vi "RealTime.vi"() -> ()   [LabVIEW 2019]
uses:
  ByteGSAPIBase/LimsTestStep/acquisitions.ctl
  <vilib>/Bytelabs/ByteChannelsSetting/ChannelSettingsLib/ChannelsRepos/ChannelsRepoXML/ChannelsRepoXML.lvclass
  C:/Program Files (x86)/National Instruments/LabVIEW 2019/vi.lib/Bytelabs/ByteChannelsSetting/ChannelSettingsLib/ChannelsRepos/ChannelsRepoBase/ChannelsRepoBase.lvclass
  TypeDef/ChannelInfo.ctl
  ByteGSAPIBase/ByteGSAPIBase.lvclass
  TypeDef/TCPMessage.ctl
  <vilib>/Bytelabs/ByteChannelsSetting/ChannelSettingsLib/ChannelsClasses/ChannelBase/ChannelBase.lvclass/ChannelBase.ctl
  ByteGSAPIBase/UpdateChannelsList/fields.ctl
  ByteGSAPIBase/TypeDef/Step.ctl
  ByteGSAPIBase/TypeDef/Asset.ctl
  <vilib>/Utility/xml.llb/Write to XML File(string).vi
  bytetcp/TCPLib/TCP_Class/TCP.lvclass
  <vilib>/Bytelabs/ByteSimpleQ/ByteSimpleQ/ByteSimpleQ.lvlib
  <vilib>/Bytelabs/ByteChannelsSetting/ChannelSettingsLib/ChannelsRepos/ChannelsRepoBase/ChannelsRepoBase.lvclass
  <vilib>/Bytelabs/ByteChannelsSetting/ChannelSettingsLib/ChannelsClasses/ChannelBase/ChannelBase.lvclass
panel:
  out "error out":errorcluster
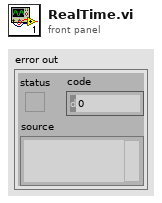
[diagram p1: front panel]
types:
  T1 = typedef "ChannelInfo.ctl" = cluster{"Tag":string, "HW Resource":string, "Raw":dbl}
  T2 = typedef "ByteGSWebAPI.lvlib/ByteGSAPIBase.lvclass/acquisitions.ctl" = cluster{"tags":cluster{"step_id":i32, "test_slug":string, "asset_slug":string}, "acquisitions":cluster{"timestamp":string, "fields":cluster{"name":string, "value":dbl}[]}[]}
  T3 = cluster{"queue out":refnum<queue>, "Acquisitions":T2, "Info":T1[], "TCP_Class":refnum<class "TCP.lvclass">, "Continous?":bool, "Duration":dbl, "ByteGSAPIBase in":refnum<class "ByteGSAPIBase.lvclass">}
  T4 = cluster{"ByteGSAPIBase in":refnum<class "ByteGSAPIBase.lvclass">, "TCP_Class":refnum<class "TCP.lvclass">, "ChannelsRepoBase out":refnum<class "ChannelsRepoXML.lvclass">, "queue out":refnum<queue>}
  T5 = cluster{"ChannelsRepoBase out":refnum<class "ChannelsRepoXML.lvclass">, "channels":string[], "Duration":dbl, "id":i32, "prova.slug":string, "Continous?":bool, "ByteGSAPIBase in":refnum<class "ByteGSAPIBase.lvclass">}
  T6 = cluster{"timestamp":string, "fields":cluster{"name":string, "value":dbl}[]}
  T7 = typedef "TCPMessage.ctl" = cluster{"Message":string, "Data":variant}
  T8 = cluster{"timestamp":string, "fields":cluster{"name":string, "value":dbl}[]}[]
  T9 = typedef "ByteGSWebAPI.lvlib/ByteGSAPIBase.lvclass/fields.ctl" = cluster{"asset_slug":string, "fields":string[]}
  T10 = typedef "ByteGSWebAPI.lvlib/ByteGSAPIBase.lvclass/Step.ctl" = cluster{"id":i32, "descrizione":string, "prova":cluster{"slug":string}, "assets":T11[], "criterio_accettazione":string, "valore_criterio_accettazione_max":dbl, "valore_criterio_accettazione_min":dbl, "udm_criterio_accettazione":string, "duration_prova":string, "udm_duration_prova":string, "valore_prova":dbl, "ordine":i32, "user":i32, "link_automation":string, "instruction_automation":string, "data_completamento_checklist":timestamp, "outcome":bool, "step_type":string, "channels":string[]}
  T11 = typedef "ByteGSWebAPI.lvlib/ByteGSAPIBase.lvclass/Asset.ctl" = cluster{"descrizione":string, "slug":string, "id":i32}
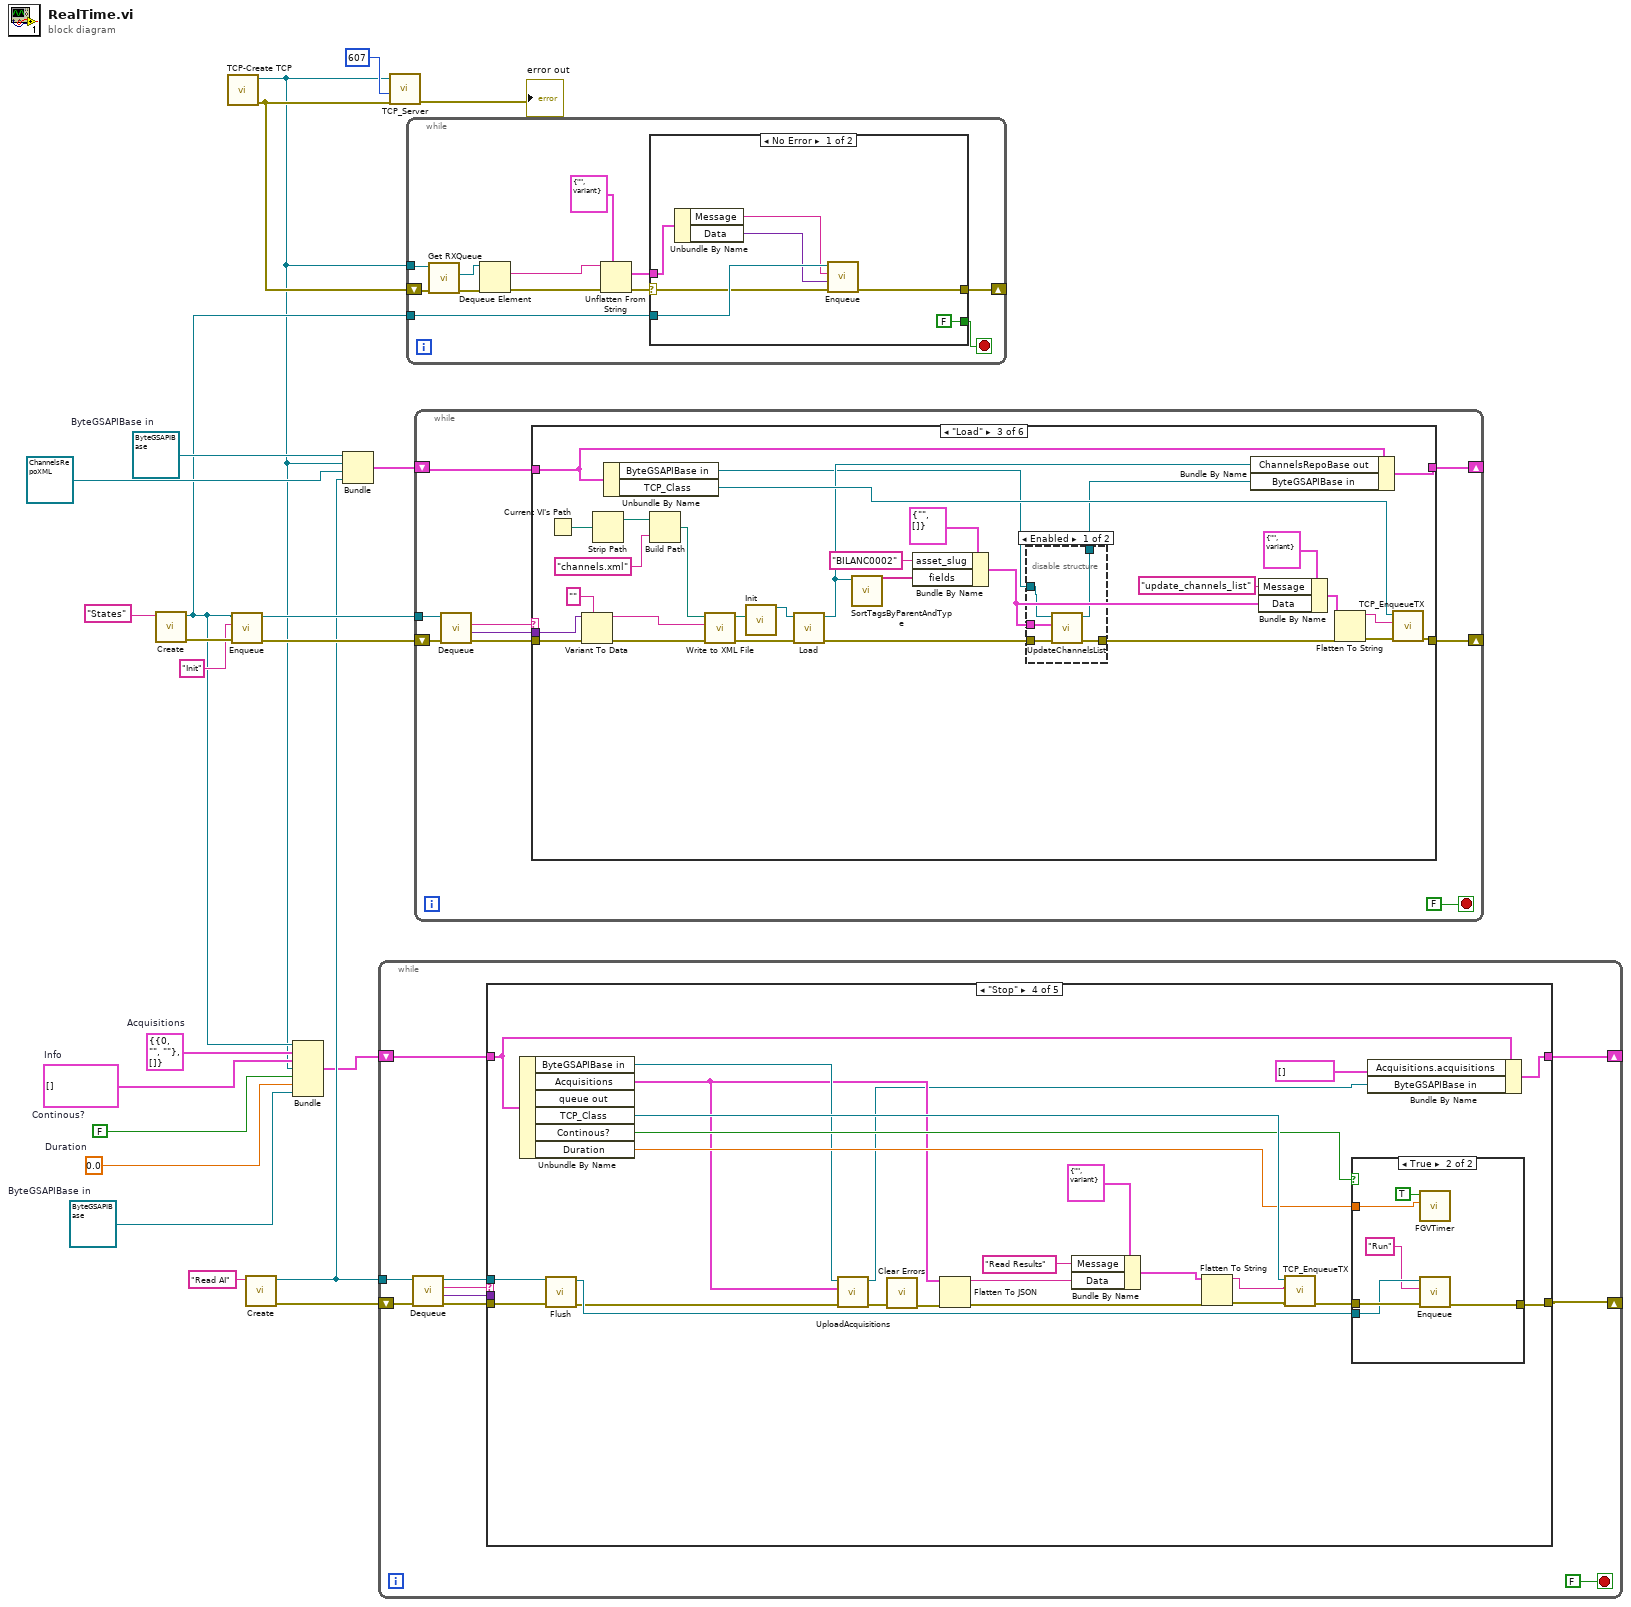
[diagram p0: block diagram]
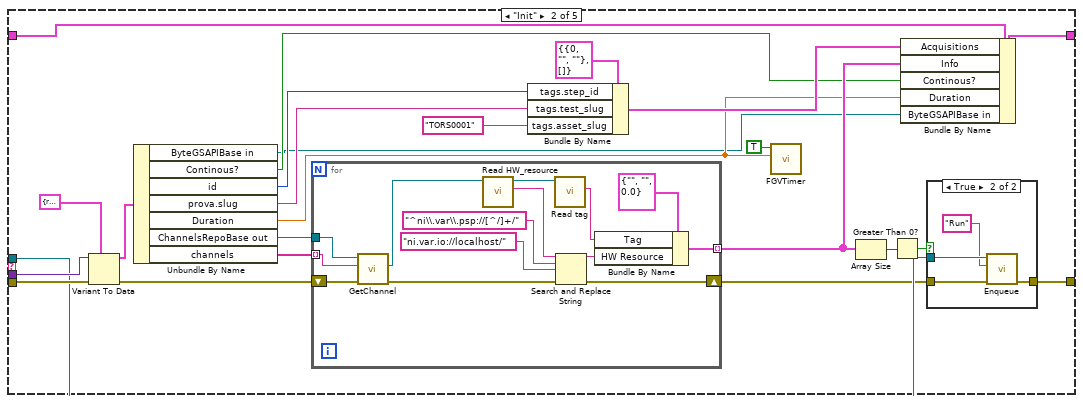
[diagram p3: hidden frame]
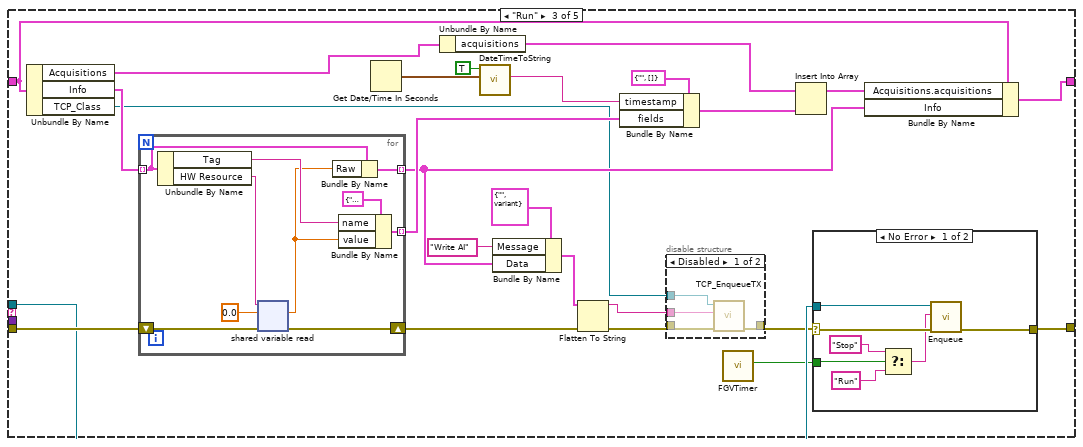
[diagram p5: hidden frame]
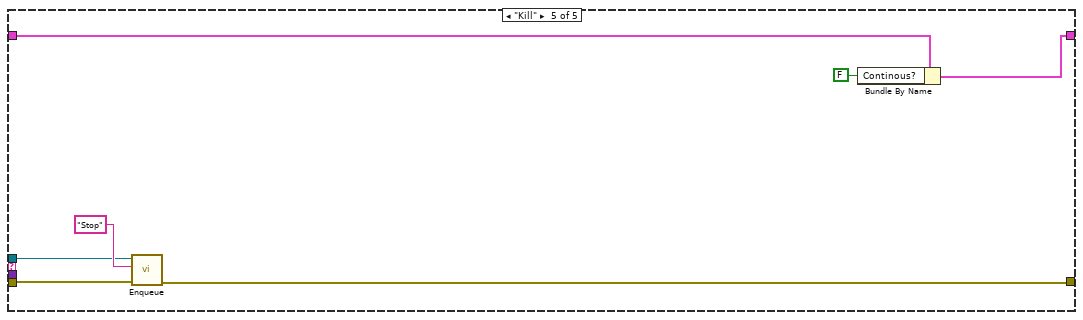
[diagram p9: hidden frame]
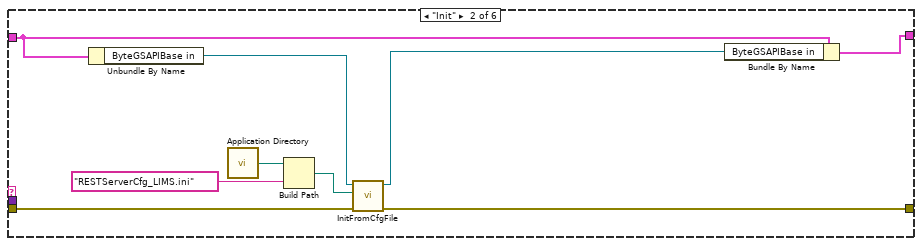
[diagram p11: hidden frame]
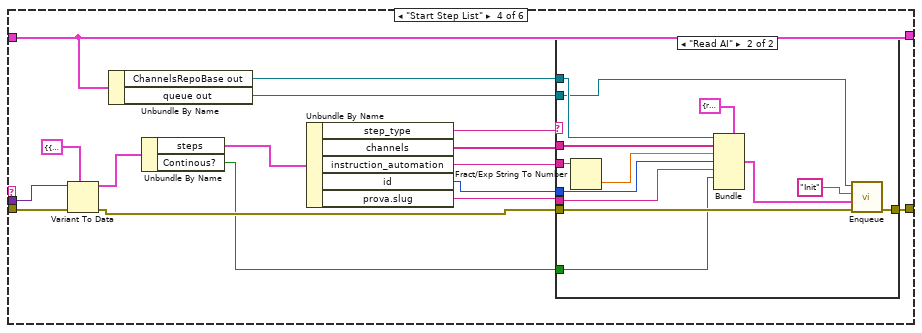
[diagram p13: hidden frame]
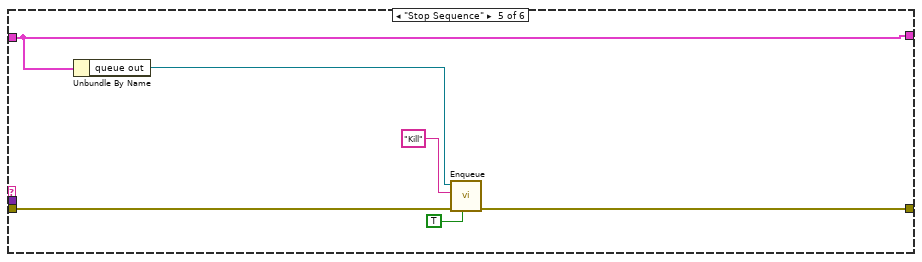
[diagram p15: hidden frame]
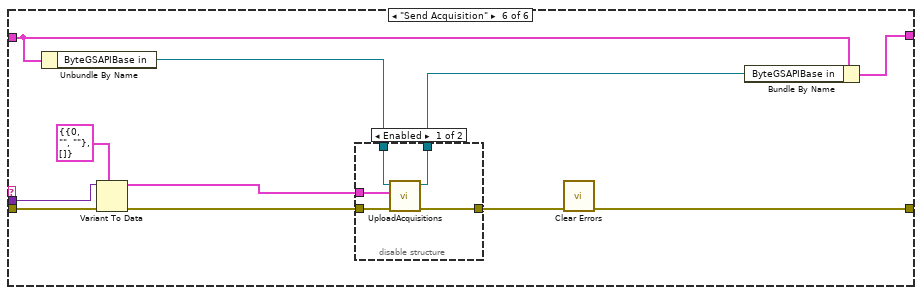
[diagram p16: hidden frame]
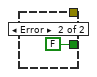
[diagram p18: hidden frame]
diagram:
  w1 = refnum<class "ByteGSAPIBase.lvclass"> refnum  # ByteGSAPIBase in
  w2 = 0.0  # Duration
  w3 = FALSE  # Continous?
  w6 = T1[] []  # Info
  w7 = T2 {"tags"={"step_id"=0, "test_slug"="", "asset_slug"=""}, "acquisitions"=[]}  # Acquisitions
  w12 = refnum<class "ByteGSAPIBase.lvclass"> refnum  # ByteGSAPIBase in
  n1 = call <vilib>:"Create.vi"("name (unnamed)"="States") -> ("error out"=w16:errorcluster, "queue out"=w8:refnum<queue>)  [unwired: 8 in, 1 out]
  n2 = call "TCP-Create TCP.vi"() -> ("error out"=w22:errorcluster, "TCP_Class"=w5:refnum<class "TCP.lvclass">)  [unwired: 9 in, 1 out]
  n3 = call <vilib>:"Enqueue.vi"("error in (no error)"=w16, "message"="Init", "queue in"=w8) -> ("error out"=w15:errorcluster, "queue out"=w14:refnum<queue>)  [unwired: 6 in, 1 out]
  n4 = call <vilib>:"Create.vi"("name (unnamed)"="Read AI") -> ("error out"=w18:errorcluster, "queue out"=w10:refnum<queue>)  [unwired: 8 in, 1 out]
  n5 = Bundle("queue out"=w8, "Acquisitions"=w7, "Info"=w6, "TCP_Class"=w5, "Continous?"=w3, "Duration"=w2, "ByteGSAPIBase in"=w1) -> (w4:T3)  [unwired: 1 in]
  n6 = Bundle("ByteGSAPIBase in"=w12, "TCP_Class"=w5, "ChannelsRepoBase out"=refnum<class "ChannelsRepoXML.lvclass"> refnum, "queue out"=w10) -> (w9:T4)  [unwired: 1 in]
  n7 = while {
    tunnel: w10 -> [w32]
    shift-right: [w26] -> _
    shift-left: w18 -> [w31]
    shift-right: [w23] -> _
    shift-left: w4 -> [w24]
    stop <- FALSE stop-if-true
    n8 = call <vilib>:"Dequeue.vi"("error in (no error)"=w31, "queue in"=w32) -> ("error out"=w30:errorcluster, "data"=w28:variant, "message"=w29:string, "queue out"=w27:refnum<queue>)  [unwired: 5 in, 1 out]
    n9 = case shown="\"Stop\"" w29 {
      tunnel: w30 -> [w34 w58 w102 w148 w161]
      tunnel: w28 -> [_ w57 _ _ _]
      tunnel: w27 -> [_ w53 w101 w147 w160]
      tunnel: [w34 w52 w100 w136 w159] -> w26
      tunnel: w24 -> [w33 w43 w81 w133 w158]
      tunnel: [w33 w41 w79 w132 w156] -> w23
      frame Default {
      }
      frame "Init" {
        n10 = Variant To Data(error in=w58, type=T5 {"ChannelsRepoBase out"=refnum, "channels"=[], "Duration"=0.0, "id"=0, "prova.slug"="", "Continous?"=FALSE, "ByteGSAPIBase in"=refnum} ("output cluster"), Variant=w57) -> (data=w51:T5, error out=w56:errorcluster)
        n11 = Unbundle By Name(w51) -> ("ByteGSAPIBase in"=w35:refnum<class "ByteGSAPIBase.lvclass">, "Continous?"=w39:bool, "id"=w45:i32, "prova.slug"=w44:string, "Duration"=w37:dbl, "ChannelsRepoBase out"=w49:refnum<class "ChannelsRepoXML.lvclass">, "channels"=w50:string[])
        n12 = for {
          shift-right: [w72] -> w48
          shift-left: w56 -> [w67]
          tunnel: [w69] -> w40 mode=indexing
          tunnel: w50 -> [w65] mode=indexing
          tunnel: w49 -> [w68]
          n13 = call <vilib>:"GetChannel.vi"("error in (no error)"=w67, "tag"=w65, "ChannelsRepoBase in"=w68) -> ("error out"=w66:errorcluster, "channel"=w64:refnum<class "ChannelBase.lvclass">)  [unwired: 5 in, 2 out]
          n14 = call <vilib>:"Read HW_resource.vi"("ChannelBase in"=w64) -> ("HW_resource"=w77:string, "ChannelBase out"=w74:refnum<class "ChannelBase.lvclass">)  [unwired: 9 in]
          n15 = call <vilib>:"Read tag.vi"("ChannelBase in"=w74) -> ("tag"=w73:string)  [unwired: 9 in, 1 out]
          n16 = Search and Replace String(input string=w77, search string="^ni\\.var\\.psp://[^/]+/", replace string="ni.var.io://localhost/" ("replace string (\"\")"), error in=w66) -> (result string=w71:string, error out=w72:errorcluster)  [unwired: 4 in, 2 out]
          n17 = Bundle By Name(cluster=T1 {"Tag"="", "HW Resource"="", "Raw"=0.0} ("output cluster"), "Tag"=w73, "HW Resource"=w71) -> (w69:T1)
        }
        n18 = Bundle By Name(cluster=T2 {"tags"={"step_id"=0, "test_slug"="", "asset_slug"=""}, "acquisitions"=[]} ("Cluster"), "tags.step_id"=w45, "tags.test_slug"=w44, "tags.asset_slug"="TORS0001") -> (w42:T2)
        n19 = call "FGVTimer.vi"("set timer"=w37, "Reset"=TRUE) -> ()  [unwired: 8 in, 2 out]
        n20 = Array Size(array=w40) -> (size(s)=w55:i32)
        n21 = Greater Than 0?(x=w55) -> (x > 0?=w54:bool)
        n22 = Bundle By Name(cluster=w43, "Acquisitions"=w42, "Info"=w40, "Continous?"=w39, "Duration"=w37, "ByteGSAPIBase in"=w35) -> (w41:T3)
        n23 = case shown="True" w54 {
          tunnel: w53 -> [_ w63]
          tunnel: [w59 w61] -> w52
          tunnel: w48 -> [w59 w60]
          frame False {
          }
          frame True {
            n24 = call <vilib>:"Enqueue.vi"("error in (no error)"=w60, "message"="Run", "queue in"=w63) -> ("error out"=w61:errorcluster)  [unwired: 6 in, 2 out]
          }
        }
      }
      frame "Run" {
        n25 = Unbundle By Name(w81) -> ("Acquisitions"=w82:T2, "Info"=w83:T1[], "TCP_Class"=w78:refnum<class "TCP.lvclass">)
        n26 = for {
          shift-right: [w120] -> w89
          shift-left: w102 -> [w124]
          tunnel: w83 -> [w121] mode=indexing
          tunnel: [w119] -> w80 mode=indexing
          tunnel: [w116] -> w95 mode=indexing
          n27 = Unbundle By Name(w121) -> ("Tag"=w117:string, "HW Resource"=w122:string)
          n28 = shared-variable-read(w122, w124, 0.0) -> (w120:errorcluster, w115:dbl)  [unwired: 2 out]
          n29 = Bundle By Name(cluster=w121, "Raw"=w115) -> (w119:T1)
          n30 = Bundle By Name(cluster=cluster{"name":string, "value":dbl} {"name"="", "value"=0.0} ("fields"), "name"=w117, "value"=w115) -> (w116:cluster{"name":string, "value":dbl})
        }
        n31 = Get Date/Time In Seconds() -> (seconds since 1Jan1904=w86:timestamp)
        n32 = Unbundle By Name(w82) -> ("acquisitions"=w93:T8)
        n33 = call "DateTimeToString.vi"("current time"=w86, "include Time?"=TRUE) -> ("date string"=w85:string)  [unwired: 8 in, 1 out]
        n34 = Bundle By Name(cluster=T7 {"Message"="", "Data"=variant}, "Message"="Write AI", "Data"=w80) -> (w98:T7)
        n35 = Flatten To String(anything=w98, error in (no error)=w89) -> (data string=w90:string, error out=w91:errorcluster)  [unwired: 2 in, 1 out]
        n36 = Bundle By Name(cluster=T6 {"timestamp"="", "fields"=[]} ("acquisition"), "timestamp"=w85, "fields"=w95) -> (w94:T6)
        n37 = disable-structure shown="Disabled" {
          disable-tunnel: w91 -> [w106 _]
          disable-tunnel: w90 -> [w105 _]
          disable-tunnel: [w104 _] -> w87
          disable-tunnel: w78 -> [w103 _]
          frame Disabled {
            n38 = call-dynamic "TCP_EnqueueTX.vi"("error in (no error)"=w106, "Msg to Transmit"=w105, "TCP in"=w103) -> ("error out"=w104:errorcluster)  [unwired: 7 in, 1 out]
          }
          frame Enabled {
          }
        }
        n39 = call "FGVTimer.vi"() -> ("Elapsed?"=w88:bool)  [unwired: 10 in, 1 out]
        n40 = Insert Into Array(array=w93, new element=w94) -> (w92:T8)  [unwired: 1 in]
        n41 = case shown="No Error" w87 {
          selector: w87 -> [w113 w114]
          tunnel: w101 -> [w111 _]
          tunnel: [w112 w114] -> w100
          tunnel: w88 -> [w110 _]
          frame No Error {
            n42 = Select(t="Stop" ("message"), s=w110, f="Run" ("message")) -> (s? t:f=w107:string)
            n43 = call <vilib>:"Enqueue.vi"("error in (no error)"=w113, "message"=w107, "queue in"=w111) -> ("error out"=w112:errorcluster)  [unwired: 6 in, 2 out]
          }
          frame Error {
          }
        }
        n44 = Bundle By Name(cluster=w81, "Acquisitions.acquisitions"=w92, "Info"=w80) -> (w79:T3)
      }
      frame "Stop" {
        n45 = Unbundle By Name(w133) -> ("ByteGSAPIBase in"=w129:refnum<class "ByteGSAPIBase.lvclass">, "Acquisitions"=w128:T2, "TCP_Class"=w139:refnum<class "TCP.lvclass">, "Continous?"=w138:bool, "Duration"=w134:dbl)  [unwired: 1 out]
        n46 = call <vilib>:"Flush.vi"("error in"=w148, "queue in"=w147) -> ("error out"=w130:errorcluster, "queue out"=w135:refnum<queue>)  [unwired: 8 in]
        n47 = call-dynamic "UploadAcquisitions.vi"("error in (no error)"=w130, "Acquisitions"=w128, "ByteGSAPIBase in"=w129) -> ("error out"=w126:errorcluster, "ByteGSAPIBase out"=w127:refnum<class "ByteGSAPIBase.lvclass">)  [unwired: 7 in]
        n48 = call <vilib>:"Clear Errors.vi"("error in (no error)"=w126) -> ("error out"=w125:errorcluster)  [unwired: 5 in, 1 out]
        n49 = Flatten To JSON(anything=w128, error in (no error)=w125) -> (JSON string=w140:string, 11:w141:errorcluster)  [unwired: 1 in]
        n50 = Bundle By Name(cluster=T7 {"Message"="", "Data"=variant}, "Message"="Read Results", "Data"=w140) -> (w145:T7)
        n51 = Flatten To String(anything=w145, error in (no error)=w141) -> (data string=w142:string, error out=w143:errorcluster)  [unwired: 2 in, 1 out]
        n52 = call-dynamic "TCP_EnqueueTX.vi"("error in (no error)"=w143, "Msg to Transmit"=w142, "TCP in"=w139) -> ("error out"=w137:errorcluster)  [unwired: 7 in, 1 out]
        n53 = case shown="True" w138 {
          tunnel: w137 -> [w149 w155]
          tunnel: [w149 w154] -> w136
          tunnel: w135 -> [_ w153]
          tunnel: w134 -> [_ w150]
          frame False {
          }
          frame True {
            n54 = call "FGVTimer.vi"("set timer"=w150, "Reset"=TRUE) -> ()  [unwired: 8 in, 2 out]
            n55 = call <vilib>:"Enqueue.vi"("error in (no error)"=w155, "message"="Run", "queue in"=w153) -> ("error out"=w154:errorcluster)  [unwired: 6 in, 2 out]
          }
        }
        n56 = Bundle By Name(cluster=w133, "Acquisitions.acquisitions"=T8 [], "ByteGSAPIBase in"=w127) -> (w132:T3)
      }
      frame "Kill" {
        n57 = call <vilib>:"Enqueue.vi"("error in (no error)"=w161, "message"="Stop", "queue in"=w160) -> ("error out"=w159:errorcluster)  [unwired: 6 in, 2 out]
        n58 = Bundle By Name(cluster=w158, "Continous?"=FALSE) -> (w156:T3)
      }
    }
  }
  n59 = call "TCP_Server.vi"("error in (no error)"=w22, "TxPort"=u16 607, "TCP.lvlib:TCP.lvclass"=w5) -> ("error out"=→"error out":errorcluster)  [unwired: 8 in]
  n60 = while {
    tunnel: w5 -> [w166]
    tunnel: w8 -> [w174]
    shift-right: [w170] -> _
    shift-left: w22 -> [w167]
    stop <- w163 stop-if-true
    # "Receiver"
    n61 = call-dynamic "Get RXQueue.vi"("error in (no error)"=w167, "TCP in"=w166) -> ("error out"=w169:errorcluster, "RX"=w168:refnum<queue>)  [unwired: 7 in, 1 out]
    n62 = Dequeue Element(queue=w168, error in (no error)=w169) -> (element=w164:string, error out=w165:errorcluster)  [unwired: 1 in, 2 out]
    n63 = Unflatten From String(type=T7 {"Message"="", "Data"=variant}, binary string=w164, error in (no error)=w165) -> (value=w171:T7, error out=w173:errorcluster)  [unwired: 2 in, 1 out]
    n64 = case shown="No Error" w173 {
      selector: w173 -> [w180 _]
      tunnel: w174 -> [w181 _]
      tunnel: w171 -> [w179 _]
      tunnel: [w176 _] -> w170
      tunnel: [FALSE FALSE] -> w163
      frame No Error {
        n65 = Unbundle By Name(w179) -> ("Message"=w177:string, "Data"=w178:variant)
        n66 = call <vilib>:"Enqueue.vi"("error in (no error)"=w180, "data"=w178, "message"=w177, "queue in"=w181) -> ("error out"=w176:errorcluster)  [unwired: 5 in, 2 out]
      }
      frame Error {
      }
    }
  }
  n67 = while {
    tunnel: w14 -> [w190]
    shift-right: [w185] -> _
    shift-left: w15 -> [w191]
    shift-right: [w183] -> _
    shift-left: w9 -> [w184]
    stop <- FALSE stop-if-true
    n68 = call <vilib>:"Dequeue.vi"("error in (no error)"=w191, "queue in"=w190) -> ("error out"=w189:errorcluster, "data"=w188:variant, "message"=w187:string)  [unwired: 5 in, 2 out]
    n69 = case shown="\"Load\"" w187 {
      tunnel: w189 -> [w193 w202 w224 w254 w273 w285]
      tunnel: w188 -> [_ _ w223 w253 _ w284]
      tunnel: [w193 w201 w218 w250 w272 w279] -> w185
      tunnel: w184 -> [w192 w196 w211 w246 w270 w277]
      tunnel: [w192 w194 w210 w246 w270 w276] -> w183
      frame Default {
      }
      frame "Init" {
        n70 = Unbundle By Name(w196) -> ("ByteGSAPIBase in"=w197:refnum<class "ByteGSAPIBase.lvclass">)
        n71 = call <vilib>:"Application Directory.vi"() -> ("Application Directory"=w199:path)
        n72 = Build Path(base path=w199, name or relative path="RESTServerCfg_LIMS.ini") -> (appended path=w198:path)
        n73 = call-dynamic "InitFromCfgFile.vi"("error in (no error)"=w202, "configuration file path"=w198, "ByteGSAPIBase in"=w197) -> ("error out"=w201:errorcluster, "ByteGSAPIBase out"=w195:refnum<class "ByteGSAPIBase.lvclass">)  [unwired: 7 in]
        n74 = Bundle By Name(cluster=w196, "ByteGSAPIBase in"=w195) -> (w194:T4)
      }
      frame "Load" {
        n75 = Current VI's Path() -> (path=w228:path)
        n76 = Variant To Data(error in=w224, type="", Variant=w223) -> (data=w231:string, error out=w230:errorcluster)
        n77 = Strip Path(path=w228) -> (stripped path=w227:path)  [unwired: 1 out]
        n78 = Unbundle By Name(w211) -> ("ByteGSAPIBase in"=w206:refnum<class "ByteGSAPIBase.lvclass">, "TCP_Class"=w212:refnum<class "TCP.lvclass">)
        n79 = Build Path(base path=w227, name or relative path="channels.xml") -> (appended path=w226:path)
        n80 = call-poly <vilib>:"Write to XML File.vi"("error in (no error)"=w230, "XML Input"=w231, "XML File Path"=w226) -> ("error out"=w222:errorcluster, "XML File Path(duplicate)"=w225:path)  [unwired: 6 in, 1 out]
        n81 = call <vilib>:"Init.vi"("XML file path"=w225) -> ("ChannelsRepoXML out"=w221:refnum<class "ChannelsRepoXML.lvclass">)  [unwired: 10 in]
        n82 = call <vilib>:"Load.vi"("error in (no error)"=w222, "ChannelsRepoBase in"=w221) -> ("error out"=w208:errorcluster, "ChannelsRepoBase out"=w209:refnum<class "ChannelsRepoXML.lvclass">)  [unwired: 7 in, 1 out]
        n83 = call <vilib>:"SortTagsByParentAndType.vi"("ChannelsRepoBase in"=w209) -> ("sorted tags"=w219:string[])  [unwired: 8 in, 2 out]
        n84 = Bundle By Name(cluster=T9 {"asset_slug"="", "fields"=[]} ("Channels"), "asset_slug"="BILANC0002", "fields"=w219) -> (w205:T9)
        n85 = disable-structure shown="Enabled" {
          disable-tunnel: w208 -> [w237 _]
          disable-tunnel: [w236 _] -> w207
          disable-tunnel: w206 -> [w235 w238]
          disable-tunnel: w205 -> [w234 _]
          disable-tunnel: [w233 w238] -> w204
          frame Enabled {
            n86 = call "UpdateChannelsList.vi"("error in (no error)"=w237, "Channels"=w234, "ByteGSAPIBase in"=w235) -> ("error out"=w236:errorcluster, "ByteGSAPIBase out"=w233:refnum<class "ByteGSAPIBase.lvclass">)  [unwired: 7 in]
          }
          frame Disabled {
          }
        }
        n87 = Bundle By Name(cluster=w211, "ChannelsRepoBase out"=w209, "ByteGSAPIBase in"=w204) -> (w210:T4)
        n88 = Bundle By Name(cluster=T7 {"Message"="", "Data"=variant} ("Cluster"), "Message"="update_channels_list", "Data"=w205) -> (w214:T7)
        n89 = Flatten To String(anything=w214, error in (no error)=w207) -> (data string=w213:string, error out=w215:errorcluster)  [unwired: 2 in, 1 out]
        n90 = call-dynamic "TCP_EnqueueTX.vi"("error in (no error)"=w215, "Msg to Transmit"=w213, "TCP in"=w212) -> ("error out"=w218:errorcluster)  [unwired: 7 in, 1 out]
      }
      frame "Start Step List" {
        n91 = Variant To Data(error in=w254, type=cluster{"steps":T10, "Continous?":bool} {"steps"={"id"=0, "descrizione"="", "prova"={"slug"=""}, "assets"=[], "criterio_accettazione"="", "valore_criterio_accettazione_max"=0.0, "valore_criterio_accettazione_min"=0.0, "udm_criterio_accettazione"="", "duration_prova"="", "udm_duration_prova"="", "valore_prova"=0.0, "ordine"=0, "user"=0, "link_automation"="", "instruction_automation"="", "data_completamento_checklist"=timestamp(0 s since 1904-01-01), "outcome"=FALSE, "step_type"="", "channels"=[]}, "Continous?"=FALSE}, Variant=w253) -> (data=w241:cluster{"steps":T10, "Continous?":bool}, error out=w251:errorcluster)
        n92 = Unbundle By Name(w246) -> ("ChannelsRepoBase out"=w247:refnum<class "ChannelsRepoXML.lvclass">, "queue out"=w245:refnum<queue>)
        n93 = Unbundle By Name(w241) -> ("steps"=w240:T10, "Continous?"=w239:bool)
        n94 = Unbundle By Name(w240) -> ("step_type"=w252:string, "channels"=w249:string[], "instruction_automation"=w248:string, "id"=w244:i32, "prova.slug"=w243:string)
        n95 = case shown="\"Read AI\"" w252 {
          tunnel: w251 -> [w255 w268]
          tunnel: [w255 w267] -> w250
          tunnel: w249 -> [_ w265]
          tunnel: w248 -> [_ w263]
          tunnel: w247 -> [_ w260]
          tunnel: w245 -> [_ w259]
          tunnel: w244 -> [_ w258]
          tunnel: w243 -> [_ w257]
          tunnel: w239 -> [_ w256]
          frame Default {
          }
          frame "Read AI" {
            n96 = Fract/Exp String To Number(string=w263) -> (number=w262:dbl)  [unwired: 3 in, 1 out]
            n97 = Bundle(cluster=T5 {"ChannelsRepoBase out"=refnum, "channels"=[], "Duration"=0.0, "id"=0, "prova.slug"="", "Continous?"=FALSE, "ByteGSAPIBase in"=refnum} ("output cluster"), "ChannelsRepoBase out"=w260, "channels"=w265, "Duration"=w262, "id"=w258, "prova.slug"=w257, "Continous?"=w256) -> (w264:T5)  [unwired: 1 in]
            n98 = call <vilib>:"Enqueue.vi"("error in (no error)"=w268, "data"=w264, "message"="Init", "queue in"=w259) -> ("error out"=w267:errorcluster)  [unwired: 5 in, 2 out]
          }
        }
      }
      frame "Stop Sequence" {
        n99 = Unbundle By Name(w270) -> ("queue out"=w271:refnum<queue>)
        n100 = call <vilib>:"Enqueue.vi"("High priority (F)"=TRUE, "data"=w273, "message"="Kill", "queue in"=w271) -> ("error out"=w272:errorcluster)  [unwired: 5 in, 2 out]
      }
      frame "Send Acquisition" {
        n101 = Unbundle By Name(w277) -> ("ByteGSAPIBase in"=w278:refnum<class "ByteGSAPIBase.lvclass">)
        n102 = Variant To Data(error in=w285, type=T2 {"tags"={"step_id"=0, "test_slug"="", "asset_slug"=""}, "acquisitions"=[]} ("Acquisitions"), Variant=w284) -> (data=w281:T2, error out=w282:errorcluster)
        n103 = disable-structure shown="Enabled" {
          disable-tunnel: w278 -> [w290 _]
          disable-tunnel: w282 -> [w289 _]
          disable-tunnel: w281 -> [w288 _]
          disable-tunnel: [w287 _] -> w275
          disable-tunnel: [w286 _] -> w280
          frame Enabled {
            n104 = call-dynamic "UploadAcquisitions.vi"("error in (no error)"=w289, "Acquisitions"=w288, "ByteGSAPIBase in"=w290) -> ("error out"=w286:errorcluster, "ByteGSAPIBase out"=w287:refnum<class "ByteGSAPIBase.lvclass">)  [unwired: 7 in]
          }
          frame Disabled {
          }
        }
        n105 = call <vilib>:"Clear Errors.vi"("error in (no error)"=w280) -> ("error out"=w279:errorcluster)  [unwired: 5 in, 1 out]
        n106 = Bundle By Name(cluster=w277, "ByteGSAPIBase in"=w275) -> (w276:T4)
      }
    }
  }
